vi "人员信息检索.vi"(2 "工作人员编号":i32=20002, 3 "connection reference":T1) -> (0 "error out":errorcluster caption="错误输出", 1 "负责人数据":T2)   [LabVIEW 2018]
uses:
  <vilib>/addons/database/Connection.llb/Conn ObjectReference.ctl
  <vilib>/addons/database/_DB Variant To Data/Database Variant To Data.xnode
  <vilib>/addons/database/NI_Database_API.lvlib
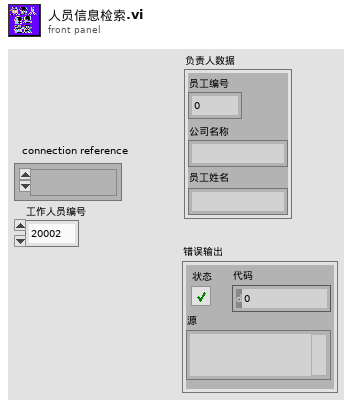
[diagram p1: front panel]
types:
  T1 = typedef "NI_Database_API.lvlib/Conn ObjectReference.ctl" = refnum<k1>
  T2 = typedef "人员信息.ctl" = cluster{"员工编号":i32, "公司名称":string, "员工姓名":string}
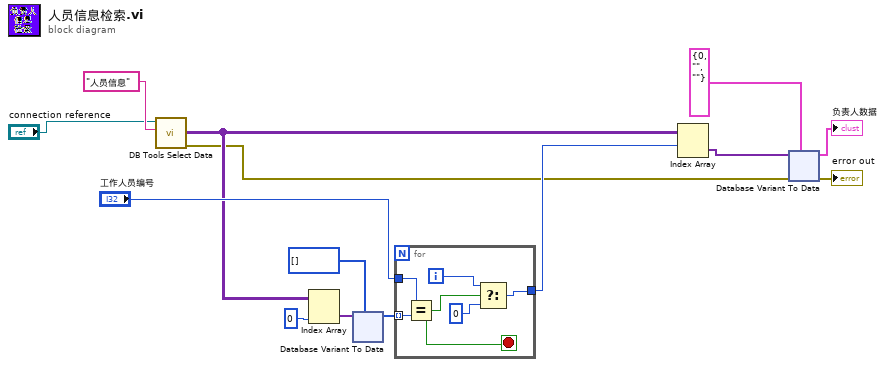
[diagram p0: block diagram]
diagram:
  n1 = call <vilib>:"DB Tools Select Data.vi"("table"="人员信息", "connection reference"="connection reference") -> ("error out"=w2:errorcluster, "data"=w7:variant[][])  [unwired: 4 in, 1 out]
  n2 = Index Array(array=w7, index (col)=0 ("禁用的索引 (列)")) -> (element=w14:variant[])  [unwired: 1 in]
  n3 = xnode "Database Variant To Data"("database variant"=w14, "type"=i32[] []) -> ("data"=w12:i32[])  [unwired: 1 in, 1 out]
  n4 = for {
    tunnel: w12 -> [w19] mode=indexing
    tunnel: "工作人员编号" -> [w20]
    tunnel: [w18] -> w10
    i -> [w16]
    stop <- w17 stop-if-true
    n5 = Equal?(x=w20, y=w19) -> (x = y?=w17:bool)
    n6 = Select(t=w16, s=w17, f=0) -> (s? t:f=w18:i32)
  }
  n7 = Index Array(array=w7, index (row)=w10) -> (element=w9:variant[])  [unwired: 1 in]
  n8 = xnode "Database Variant To Data"("database variant"=w9, "error in (no error)"=w2, "type"=T2 {"员工编号"=0, "公司名称"="", "员工姓名"=""} ("簇")) -> ("data"=→"负责人数据":T2, "error out"=→"error out":errorcluster)
